vi "ENS210_Main.vi"(8 "error in":errorcluster, 11 "Enum":T1) -> (0 "error out":errorcluster, 3 "Humidity_percent":dbl)   [LabVIEW 2016]
uses:
  ENS210_StateMachine.ctl
  <vilib>/myRIO/Instrument Drivers/Onboard IO/I2C/vis/Configure.vi
  <vilib>/myRIO/Instrument Drivers/Onboard IO/I2C/vis/Write.vi
  <vilib>/myRIO/Instrument Drivers/Onboard IO/I2C/vis/Read.vi
  <vilib>/myRIO/Instrument Drivers/Onboard IO/I2C/vis/Smart Open.vi
  <vilib>/Utility/error.llb/Error Cluster From Error Code.vi
  <vilib>/myRIO/Common/Instrument Driver Framework/myRIO v1.0/I2C/vis/myRIO v1.0 Configure I2C.vi
  <vilib>/myRIO/Common/Instrument Driver Framework/myRIO v1.0/I2C/vis/myRIO v1.0 Write I2C.vi
  <vilib>/myRIO/Common/Instrument Driver Framework/myRIO v1.0/I2C/vis/myRIO v1.0 Read I2C.vi
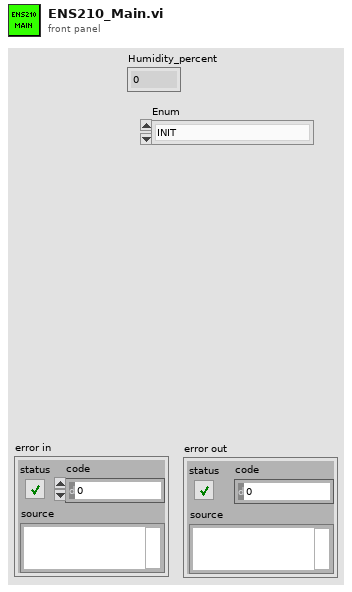
[diagram p1: front panel]
types:
  T1 = typedef "ENS210_StateMachine.ctl" = enum16{"INIT", "SET_SENSOR_MODE", "GET_SENSOR_DATA", "END", "ERROR"}
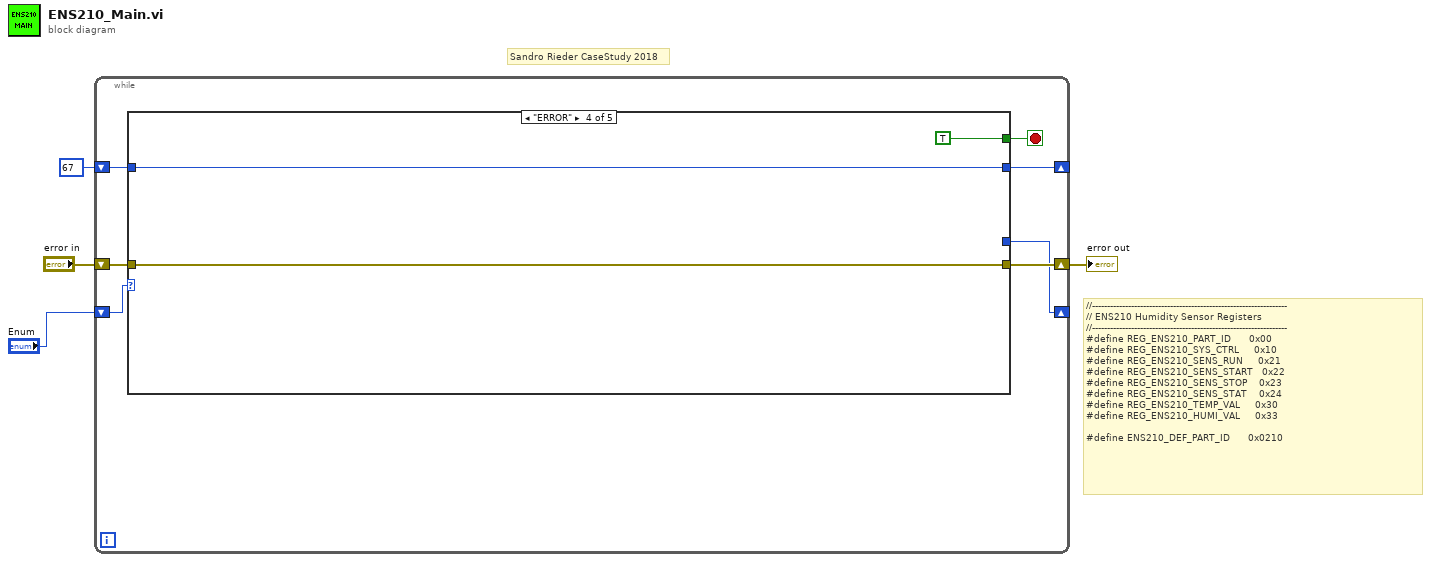
[diagram p0: block diagram]
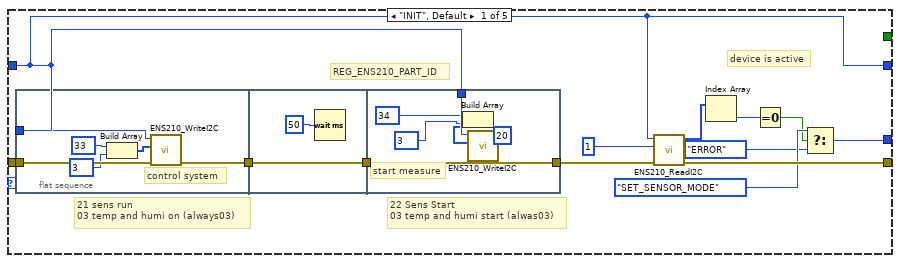
[diagram p2: hidden frame]
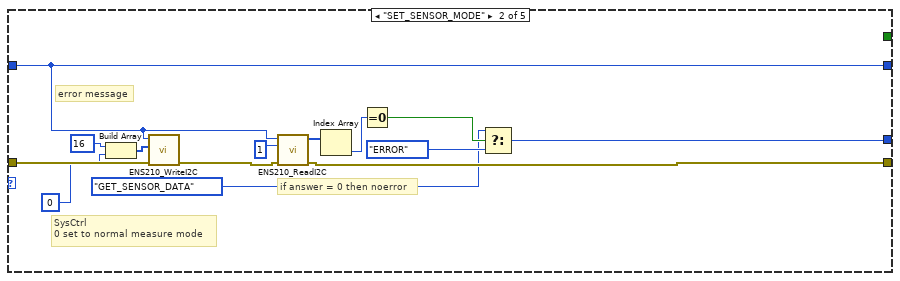
[diagram p3: hidden frame]
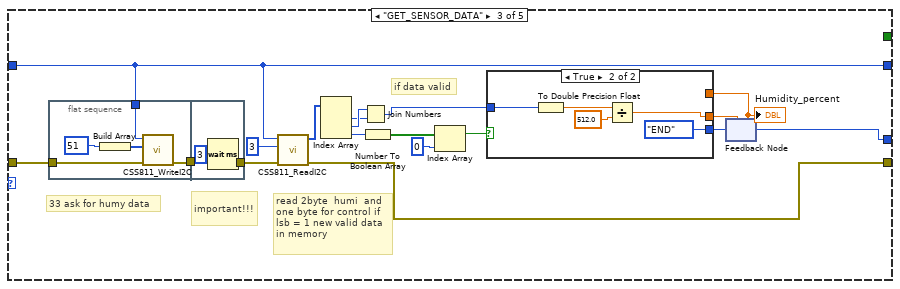
[diagram p4: hidden frame]
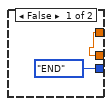
[diagram p5: hidden frame]
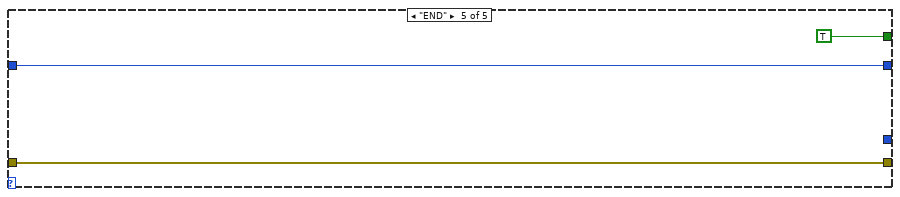
[diagram p6: hidden frame]
diagram:
  # "Sandro Rieder CaseStudy 2018"
  # "//-----------------------------------------------------------------\n// ENS210 Humidity Sensor Registers\n//-----------------------------------------------------------------\n#define REG_ENS210_PART_ID      0x00\n#define REG_ENS210_SYS_CTRL     0x10\n#define REG_ENS210_SENS_RUN     0x21\n#define REG_ENS210_SENS_START   0x22\n#define REG_ENS210_SENS_STOP    0x23\n#define REG_ENS210_SENS_STAT    0x24\n#define REG_ENS210_TEMP_VAL     0x30\n#define REG_ENS210_HUMI_VAL     0x33   \n   \n#define ENS210_DEF_PART_ID      0x0210"
  n1 = while {
    shift-right: [w8] -> _
    shift-left: u8 67 ("Slave Address (7-bit)") -> [w7]
    shift-right: [w10] -> w4
    shift-left: "error in" -> [w11]
    shift-right: [w6] -> _
    shift-left: "Enum" -> [w9]
    stop <- w5 stop-if-true
    n2 = case shown="\"ERROR\"" w9 {
      tunnel: w11 -> [w24 w44 w66 w84 w87]
      tunnel: [w22 w43 w62 w84 w87] -> w10
      tunnel: [w13 w40 w65 w85 w88] -> w8
      tunnel: w7 -> [w13 w40 w65 w85 w88]
      tunnel: [w17 w42 w64 _ _] -> w6
      tunnel: [_ _ _ TRUE TRUE] -> w5
      frame "INIT", Default {
        # "22 Sens Start\n03 temp and humi start (alwas03)"
        # "21 sens run\n03 temp and humi on (always03)"
        # "device is active"
        # "REG_ENS210_PART_ID"
        n3 = flat-sequence {
          tunnel: w24 -> [w29]
          tunnel: w13 -> [w27]
          tunnel: [w25] -> w16
          tunnel: w16 -> [w32]
          tunnel: [w32] -> w15
          tunnel: [w37] -> w14
          tunnel: w15 -> [w37]
          tunnel: w13 -> [w36]
          frame #0 {
            # "control system"
            n4 = Build Array(u8 33, u8 3) -> (w30:u8[])
            n5 = call "ENS210_WriteI2C.vi"("error in (no error)"=w29, "Bytes to Write"=w30, "Slave Address (7-bit)"=w27) -> ("error out"=w25:errorcluster)  [unwired: 6 in]
          }
          frame #1 {
            n6 = Wait (ms)(milliseconds to wait=u32 50) -> ()  [unwired: 1 out]
          }
          frame #2 {
            (unwired) u32 20 ("milliseconds to wait")
            # "start measure"
            n7 = Build Array(u8 34, u8 3) -> (w34:u8[])
            n8 = call "ENS210_WriteI2C.vi"("Bytes to Write"=w34, "Slave Address (7-bit)"=w36) -> ()  [unwired: 7 in, 1 out]
          }
        }
        n9 = call "ENS210_ReadI2C.vi"("error in (no error)"=w14, "Byte Count"=u32 1, "Slave Address (7-bit)"=w13) -> ("error out"=w22:errorcluster, "Bytes Read"=w21:u8[])  [unwired: 5 in]
        n10 = Index Array(array=w21) -> (element=w20:u8)  [unwired: 1 in]
        n11 = Equal To 0?(x=w20) -> (x = 0?=w12:bool)
        n12 = Select(t=ENS210_StateMachine."SET_SENSOR_MODE", s=w12, f=ENS210_StateMachine."ERROR") -> (s? t:f=w17:T1)
      }
      frame "SET_SENSOR_MODE" {
        # "SysCtrl\n0 set to normal measure mode"
        # "if answer = 0 then noerror"
        # "error message"
        n13 = Build Array(u8 16, u8 0) -> (w51:u8[])
        n14 = call "ENS210_WriteI2C.vi"("error in (no error)"=w44, "Bytes to Write"=w51, "Slave Address (7-bit)"=w40) -> ("error out"=w38:errorcluster)  [unwired: 6 in]
        n15 = call "ENS210_ReadI2C.vi"("error in (no error)"=w38, "Byte Count"=u32 1, "Slave Address (7-bit)"=w40) -> ("error out"=w43:errorcluster, "Bytes Read"=w48:u8[])  [unwired: 5 in]
        n16 = Index Array(array=w48) -> (element=w47:u8)  [unwired: 1 in]
        n17 = Equal To 0?(x=w47) -> (x = 0?=w46:bool)
        n18 = Select(t=ENS210_StateMachine."GET_SENSOR_DATA", s=w46, f=ENS210_StateMachine."ERROR") -> (s? t:f=w42:T1)
      }
      frame "GET_SENSOR_DATA" {
        # "read 2byte  humi  and\none byte for control if\nlsb = 1 new valid data\nin memory"
        # "33 ask for humy data"
        # "important!!!"
        # "if data valid"
        n19 = flat-sequence {
          tunnel: w66 -> [w70]
          tunnel: w65 -> [w69]
          tunnel: [w71] -> w52
          tunnel: [w75] -> w67
          tunnel: w52 -> [w75]
          frame #0 {
            n20 = Build Array(u8 51) -> (w72:u8[])
            n21 = call "CSS811_WriteI2C.vi"("error in (no error)"=w70, "Bytes to Write"=w72, "Slave Address (7-bit)"=w69) -> ("error out"=w71:errorcluster)  [unwired: 6 in]
          }
          frame #1 {
            n22 = Wait (ms)(milliseconds to wait=u32 3) -> ()  [unwired: 1 out]
          }
        }
        n23 = call "CSS811_ReadI2C.vi"("error in (no error)"=w67, "Byte Count"=u32 3, "Slave Address (7-bit)"=w65) -> ("error out"=w62:errorcluster, "Bytes Read"=w63:u8[])  [unwired: 5 in]
        n24 = Index Array(array=w63) -> (element #1=w59:u8, element #2=w60:u8, element #3=w58:u8)  [unwired: 3 in]
        n25 = Join Numbers(hi=w60, lo=w59) -> ((hi.lo)=w61:u16)
        n26 = Number To Boolean Array(number=w58) -> (Boolean array=w57:bool[])
        n27 = Index Array(array=w57, index=0) -> (element=w55:bool)
        n28 = feedback #1() -> (w53:dbl)  [unwired: 1 in]
        "Humidity_percent" <- w53
        n29 = case shown="True" w55 {
          tunnel: [ENS210_StateMachine."END" ENS210_StateMachine."END"] -> w64
          tunnel: w61 -> [_ w79]
          tunnel: [w76 w78] -> w54
          tunnel: w53 -> [w76 _]
          frame False {
          }
          frame True {
            n30 = To Double Precision Float(number=w79) -> (double precision float=w81:dbl)
            n31 = Divide(x=w81, y=512.0) -> (x/y=w78:dbl)
          }
        }
        n32 = feedback-in #1(w54) -> ()
      }
      frame "ERROR" {
      }
      frame "END" {
      }
    }
  }
  "error out" <- w4
